vi "configureTimingNow.vi"(8 "error in (no error)":errorcluster, 11 "DIO64Output in":refnum<class "DIO64Output.lvclass">) -> (0 "error out":errorcluster, 3 "DIO64Output out":refnum<class "DIO64Output.lvclass">)   [LabVIEW 2011, in "Hardware.lvlib" / "Channels.lvlib" / "DIO64Output.lvclass"]
uses:
  DIO64Output.lvclass
  DIO64Output.lvclass/DIO64Output.ctl
  <userlib>/dio64_32.LLB/DIO64 attribute value.ctl
  <userlib>/dio64_32.LLB/DIO64 attribute id.ctl
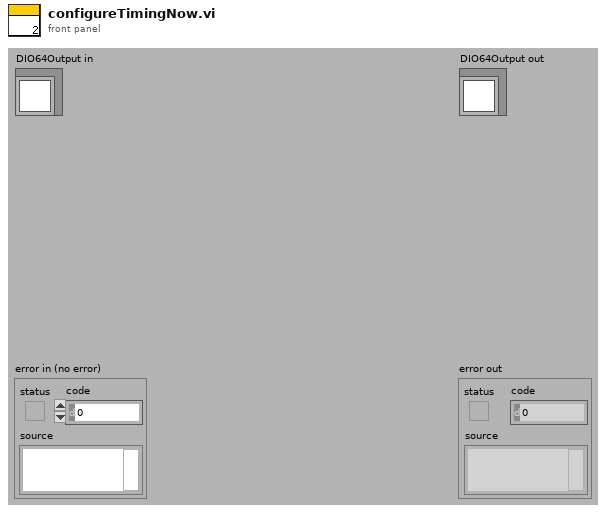
[diagram p1: front panel]
types:
  T1 = cluster{"Master Clock source":string, "Master Clock rate":dbl, "Start trigger line":string, "Scan rate":dbl, "Stop trigger line":string, "Sample Number":dbl}
  T2 = typedef "DIO64 Out Config Control.ctl" = cluster{"flags":enum16{"unused"}, "clock control":T3, "start trigger":T4, "stop trigger":T5, "DAQ clock modulo":u32, "repetitions":u32, "#transitions":u16}
  T3 = typedef "DIO64 clock control.ctl" = enum16{"internal", "external", "trig 0", "OCXO"}
  T4 = typedef "DIO64 start trig.ctl" = cluster{"source":enum16{"none", "internal", "external", "trig 2", "PXI Star"}, "type":enum16{"level", "edge", "edge to edge"}, "sense":enum16{"rising", "falling"}}
  T5 = typedef "DIO64 stop trig.ctl" = cluster{"source":enum16{"none", "internal", "external", "trig 3 in", "output FIFO"}, "type":enum16{"level", "edge"}, "sense":enum16{"falling", "rising"}}
  T6 = typedef "DIO64 attribute value.ctl" = enum16{"default", "long value", "polled", "interrupt", "packet", "demand", "local clock", "external clock", "rtsi/pxi clock", "precision clock", "20MHz", "10MHz", "precision OCXO", "enable", "disable"}
  T7 = typedef "DIO64 attribute id.ctl" = enum16{"input mode", "output mode", "input buffer size", "output buffer size", "major clock source", "input threshold percent", "output threshold percent", "input dma timeout", "rtsi/pxi global enable", "rtsi/pxi clock source", "rtsi clock/pxi trig 7 enable", "external clock enable", "pxi clock enable", "scan clock trig 0 enable", "start trig trig 2 enable", "stop trig trig 3 enable", "daq modulo trig 4 enable", "pxi star enable", "port routing", "staticOutputPorts", "serial number", "rearm enable", "SCLK enable", "FPGA info"}
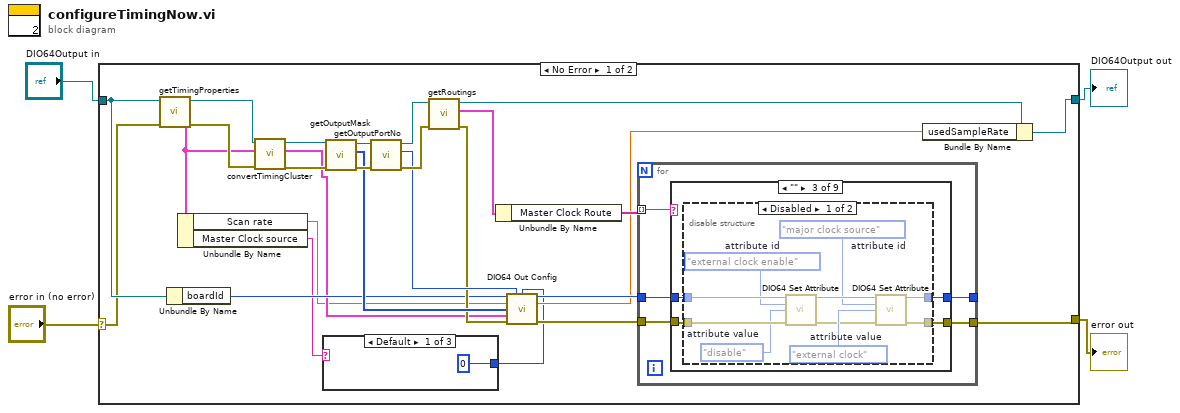
[diagram p0: block diagram]
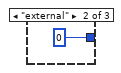
[diagram p2: hidden frame]
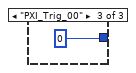
[diagram p3: hidden frame]
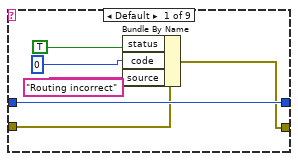
[diagram p4: hidden frame]
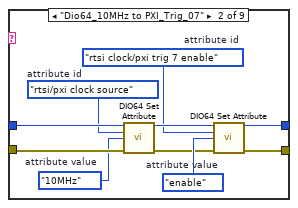
[diagram p5: hidden frame]
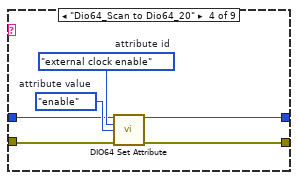
[diagram p7: hidden frame]
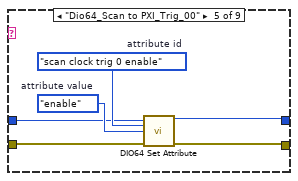
[diagram p8: hidden frame]
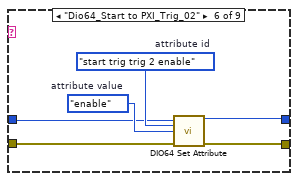
[diagram p9: hidden frame]
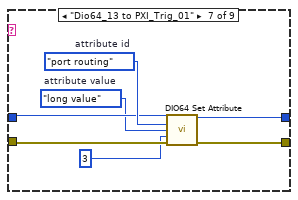
[diagram p10: hidden frame]
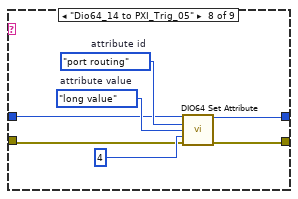
[diagram p11: hidden frame]
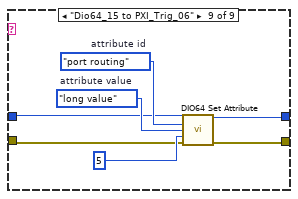
[diagram p12: hidden frame]
diagram:
  n1 = case shown="No Error" "error in (no error)" {
    selector: "error in (no error)" -> [w9 w111]
    tunnel: "DIO64Output in" -> [w11 w112]
    tunnel: [w13 w112] -> w2
    tunnel: [w23 w111] -> w1
    frame No Error {
      n2 = call-dynamic "getTimingProperties.vi"("error in (no error)"=w9, "DigitalOutput.lvclass in"=w11) -> ("error out"=w30:errorcluster, "Timing"=w18:T1, "DigitalOutput.lvclass out"=w31:refnum<class "DIO64Output.lvclass">)  [unwired: 7 in]
      n3 = Unbundle By Name(w11) -> ("boardId"=w10:i32)
      n4 = Unbundle By Name(w18) -> ("Scan rate"=w5:dbl, "Master Clock source"=w8:string)
      n5 = call "convertTimingCluster.vi"("error in (no error)"=w30, "Timing"=w18, "DIO64Output in"=w31) -> ("error out"=w26:errorcluster, "Out Config Control"=w6:T2, "DIO64Output out"=w27:refnum<class "DIO64Output.lvclass">)  [unwired: 6 in]
      n6 = case shown="Default" w8 {
        tunnel: [u32 0 ("divider") u32 0 ("divider") 0] -> w7
        frame Default {
        }
        frame "external" {
        }
        frame "PXI_Trig_00" {
        }
      }
      n7 = call "getOutputMask.vi"("error in (no error)"=w26, "DIO64Output.lvclass in"=w27) -> ("error out"=w28:errorcluster, "mask"=w19:u16[], "DIO64Output.lvclass out"=w29:refnum<class "DIO64Output.lvclass">)  [unwired: 7 in]
      n8 = call "getOutputPortNo.vi"("error in (no error)"=w28, "DIO64Output.lvclass in"=w29) -> ("error out"=w24:errorcluster, "#ports"=w20:u8, "DIO64Output.lvclass out"=w25:refnum<class "DIO64Output.lvclass">)  [unwired: 7 in]
      n9 = call-dynamic "getRoutings.vi"("error in (no error)"=w24, "DigitalOutput.lvclass in"=w25) -> ("error out"=w15:errorcluster, "Routings"=w22:cluster{"Master Clock Route":string[]}, "DigitalOutput.lvclass out"=w14:refnum<class "DIO64Output.lvclass">)  [unwired: 7 in]
      n10 = Unbundle By Name(w22) -> ("Master Clock Route"=w21:string[])
      n11 = call <userlib>:"DIO64 Out Config.vi"("board in"=w10, "#ports"=w20, "divider"=w7, "scan rate (Hz)"=w5, "mask"=w19, "Config Control"=w6, "error in (no error)"=w15) -> ("board out"=w17:u16, "actual scan rate (Hz)"=w12:dbl, "error out"=w16:errorcluster)  [unwired: 6 in]
      n12 = for {
        tunnel: [w39] -> w23
        tunnel: w16 -> [w38]
        tunnel: w17 -> [w37]
        tunnel: [w36] -> _
        tunnel: w21 -> [w35] mode=indexing
        n13 = case shown="\"\"" w35 {
          tunnel: [w43 w46 w56 w73 w78 w84 w93 w97 w105] -> w39
          tunnel: w38 -> [w44 w54 w58 w74 w80 w86 w94 w99 w106]
          tunnel: w37 -> [w45 w55 w59 w75 w81 w87 w95 w100 w107]
          tunnel: [w45 w47 w57 w72 w79 w85 w92 w98 w104] -> w36
          frame Default {
            n14 = Bundle By Name(cluster=w44, "status"=TRUE, "code"=0, "source"="Routing incorrect") -> (w43:errorcluster)
          }
          frame "Dio64_10MHz to PXI_Trig_07" {
            w49 = DIO64_attribute_value."enable"  # attribute value
            w50 = DIO64_attribute_id."rtsi clock/pxi trig 7 enable"  # attribute id
            w52 = DIO64_attribute_value."10MHz"  # attribute value
            w53 = DIO64_attribute_id."rtsi/pxi clock source"  # attribute id
            n15 = call <userlib>:"DIO64 Set Attribute.vi"("board in"=w55, "attribute id"=w53, "attribute value"=w52, "error in (no error)"=w54) -> ("board out"=w51:u16, "error out"=w48:errorcluster)  [unwired: 10 in]
            n16 = call <userlib>:"DIO64 Set Attribute.vi"("board in"=w51, "attribute id"=w50, "attribute value"=w49, "error in (no error)"=w48) -> ("board out"=w47:u16, "error out"=w46:errorcluster)  [unwired: 10 in]
          }
          frame "" {
            n17 = disable-structure shown="Disabled" {
              disable-tunnel: w59 -> [w69 w71]
              disable-tunnel: w58 -> [w68 w70]
              disable-tunnel: [w61 w71] -> w57
              disable-tunnel: [w60 w70] -> w56
              frame Disabled {
                w63 = DIO64_attribute_value."external clock"  # attribute value
                w64 = DIO64_attribute_id."major clock source"  # attribute id
                w66 = DIO64_attribute_value."disable"  # attribute value
                w67 = DIO64_attribute_id."external clock enable"  # attribute id
                n18 = call <userlib>:"DIO64 Set Attribute.vi"("board in"=w69, "attribute id"=w67, "attribute value"=w66, "error in (no error)"=w68) -> ("board out"=w65:u16, "error out"=w62:errorcluster)  [unwired: 10 in]
                n19 = call <userlib>:"DIO64 Set Attribute.vi"("board in"=w65, "attribute id"=w64, "attribute value"=w63, "error in (no error)"=w62) -> ("board out"=w61:u16, "error out"=w60:errorcluster)  [unwired: 10 in]
              }
              frame Enabled {
              }
            }
          }
          frame "Dio64_Scan to Dio64_20" {
            w76 = DIO64_attribute_value."enable"  # attribute value
            w77 = DIO64_attribute_id."external clock enable"  # attribute id
            n20 = call <userlib>:"DIO64 Set Attribute.vi"("board in"=w75, "attribute id"=w77, "attribute value"=w76, "error in (no error)"=w74) -> ("board out"=w72:u16, "error out"=w73:errorcluster)  [unwired: 10 in]
          }
          frame "Dio64_Scan to PXI_Trig_00" {
            w82 = DIO64_attribute_value."enable"  # attribute value
            w83 = DIO64_attribute_id."scan clock trig 0 enable"  # attribute id
            n21 = call <userlib>:"DIO64 Set Attribute.vi"("board in"=w81, "attribute id"=w83, "attribute value"=w82, "error in (no error)"=w80) -> ("board out"=w79:u16, "error out"=w78:errorcluster)  [unwired: 10 in]
          }
          frame "Dio64_Start to PXI_Trig_02" {
            w88 = DIO64_attribute_value."enable"  # attribute value
            w89 = DIO64_attribute_id."start trig trig 2 enable"  # attribute id
            n22 = call <userlib>:"DIO64 Set Attribute.vi"("board in"=w87, "attribute id"=w89, "attribute value"=w88, "error in (no error)"=w86) -> ("board out"=w85:u16, "error out"=w84:errorcluster)  [unwired: 10 in]
          }
          frame "Dio64_13 to PXI_Trig_01" {
            w91 = DIO64_attribute_value."long value"  # attribute value
            w96 = DIO64_attribute_id."port routing"  # attribute id
            n23 = call <userlib>:"DIO64 Set Attribute.vi"("board in"=w95, "attribute id"=w96, "attribute value"=w91, "value"=3, "error in (no error)"=w94) -> ("board out"=w92:u16, "error out"=w93:errorcluster)  [unwired: 9 in]
          }
          frame "Dio64_14 to PXI_Trig_05" {
            w102 = DIO64_attribute_value."long value"  # attribute value
            w101 = DIO64_attribute_id."port routing"  # attribute id
            n24 = call <userlib>:"DIO64 Set Attribute.vi"("board in"=w100, "attribute id"=w101, "attribute value"=w102, "value"=4, "error in (no error)"=w99) -> ("board out"=w98:u16, "error out"=w97:errorcluster)  [unwired: 9 in]
          }
          frame "Dio64_15 to PXI_Trig_06" {
            w109 = DIO64_attribute_value."long value"  # attribute value
            w108 = DIO64_attribute_id."port routing"  # attribute id
            n25 = call <userlib>:"DIO64 Set Attribute.vi"("board in"=w107, "attribute id"=w108, "attribute value"=w109, "value"=5, "error in (no error)"=w106) -> ("board out"=w104:u16, "error out"=w105:errorcluster)  [unwired: 9 in]
          }
        }
      }
      n26 = Bundle By Name(cluster=w14, "usedSampleRate"=w12) -> (w13:refnum<class "DIO64Output.lvclass">)
    }
    frame Error {
    }
  }
  "error out" <- w1
  "DIO64Output out" <- w2
